vi "Channel Load (UTF-8).vi"(7 "Wait For Load (T)":bool=TRUE, 8 "error in (no error)":errorcluster, 9 "Path":string, 10 "Channel Index":i32, 11 "Mixer in":refnum<class "Mixer.lvclass">) -> (0 "error out":errorcluster, 3 "Mixer out":refnum<class "Mixer.lvclass">)   [LabVIEW 2020, in "G-Audio.lvlib" / "Mixer.lvclass"]
doc: "Reads an audio file into memory, and associates it with a channel.\n\nWhen <b>Wait For Load</b> is true, this VI blocks until the audio file has been loaded into a channel. If <b>Wait For Load</b> is false, this VI returns immediately and the audio file is loaded asynchronously in the background. The channel will be in a Loading state while the file is read, and then set to Loaded once the load is complete, or Empty if there was an error."
uses:
  Mixer.lvclass
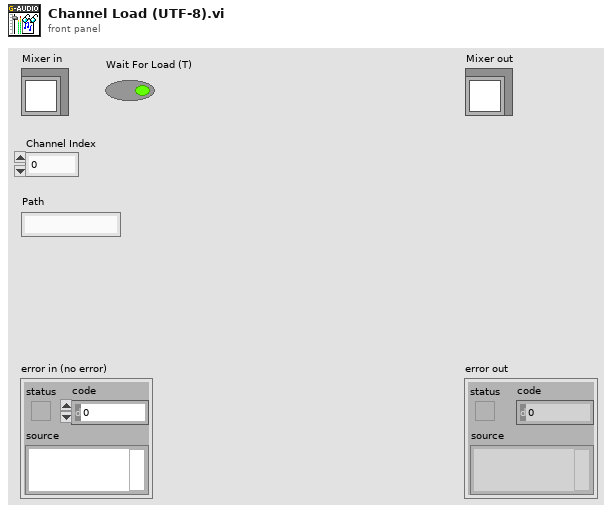
[diagram p1: front panel]
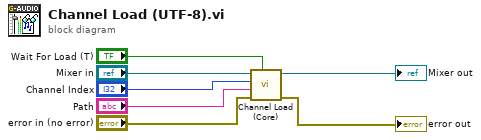
[diagram p0: block diagram]
diagram:
  n1 = call "Channel Load (Core).vi"("Wait For Load (T)"="Wait For Load (T)", "error in (no error)"="error in (no error)", "Path"="Path", "Channel Index"="Channel Index", "Mixer in"="Mixer in") -> ("error out"=→"error out":errorcluster, "Mixer out"=→"Mixer out":refnum<class "Mixer.lvclass">)  [unwired: 5 in]
